vi "AOL Z Cal-Disable Cal file load button.vi"(9 "Init":bool, 11 "Browse button ref":refnum<vi>) -> (0 "error out":errorcluster, 3 "Browse button ref":refnum<vi>)   [LabVIEW 2013]
uses:
  Typedefs/Top level VI states.ctl
  Global Variables/General Globals.vi
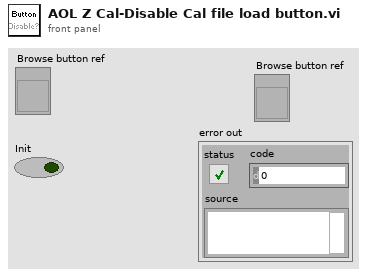
[diagram p1: front panel]
types:
  T1 = typedef "Top level VI states.ctl" = enum16{"None", "Initialise UI", "<STACK PROTOCOL STATES>", "AOL Zstack-START", "AOL Zstack-STOP", "Motor Zstack-START", "Motor Zstack-STOP", "<ACQUISITION PROTOCOL STATES> ", "Functional Acquisition-START", "Functional Acquisition-STOP", "Single Plane Acquisition-START", "Single Plane Acquisition-STOP", "Volume Acquisition-START", "Volume Acquisition-STOP", "<LIVE IMAGING PROTOCOL STATES>", "Live Imaging-START", "Live Imaging-STOP", "Live Plane Imaging-START", "Live Plane Imaging-STOP", "Live Volume Imaging-START", "Live Volume Imaging-STOP", "EXIT"}
  T2 = enum8{"Enabled", "Disabled", "Disabled and Grayed Out"}
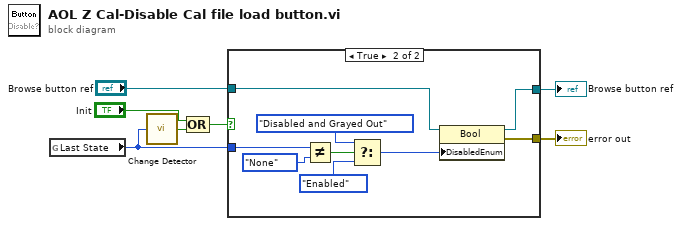
[diagram p0: block diagram]
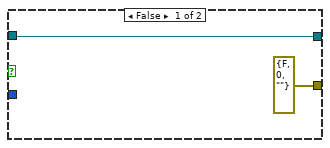
[diagram p2: hidden frame]
diagram:
  n1 = global read "General Globals.vi" "Last State"() -> (w7:T1)
  n2 = call "Change Detector.vi"("Value"=w7) -> ("Changed?"=w3:bool)
  n3 = Compound Arithmetic op=OR("Init", w3) -> (w5:bool)
  n4 = case shown="True" w5 {
    tunnel: "Browse button ref" -> [w8 w11]
    tunnel: w7 -> [_ w17]
    tunnel: [errorcluster {"status"=FALSE, "code"=0, "source"=""} ("error out") w12] -> w2
    tunnel: [w8 w10] -> w1
    frame False {
    }
    frame True {
      n5 = Not Equal?(x=w17, y=Top_level_VI_states."None" ("Last State")) -> (x != y?=w16:bool)
      n6 = Select(t=T2."Disabled and Grayed Out" ("Disabled"), s=w16, f=T2."Enabled" ("Disabled")) -> (s? t:f=w15:T2)
      n7 = property class="Bool"(reference=w11, "DisabledEnum"=w15) -> (reference out=w10:refnum<vi>, error out=w12:errorcluster)  [unwired: 1 in]
    }
  }
  "error out" <- w2
  "Browse button ref" <- w1
